vi "Parse Notes.vi"(8 "error in":errorcluster, 11 "String":string) -> (0 "error out":errorcluster, 1 "Done Reading?":bool, 2 "sr note out":string[](array[string]), 3 "result string out":string)   [LabVIEW 2018]
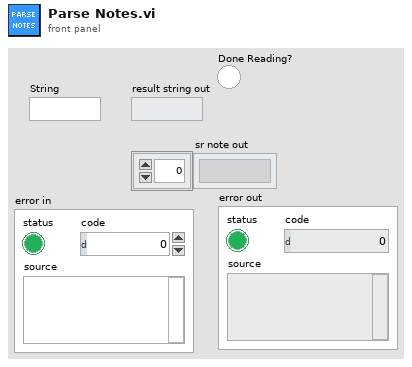
[diagram p1: front panel]
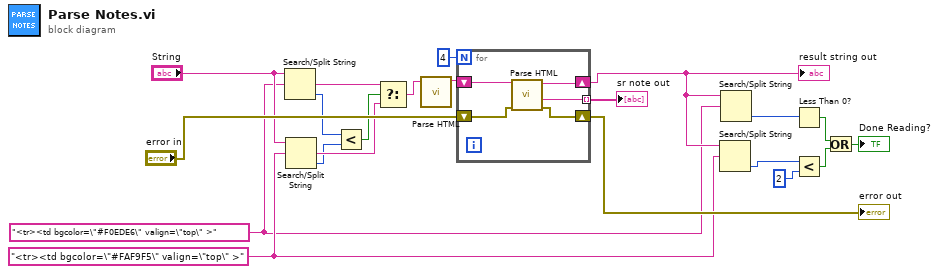
[diagram p0: block diagram]
diagram:
  w6 = "<tr><td bgcolor=\"#FAF9F5\" valign=\"top\" >" ("search string/char (-)")
  w4 = "<tr><td bgcolor=\"#F0EDE6\" valign=\"top\" >" ("search string/char (-)")
  n1 = Search/Split String(string="String", search string/char (-)=w4) -> (match + rest of string=w15:string, offset of match=w13:i32)  [unwired: 1 in, 1 out]
  n2 = Search/Split String(string="String", search string/char (-)=w6) -> (match + rest of string=w14:string, offset of match=w12:i32)  [unwired: 1 in, 1 out]
  n3 = Less?(x=w13, y=w12) -> (x < y?=w11:bool)
  n4 = Select(t=w15, s=w11, f=w14) -> (s? t:f=w3:string)
  n5 = call "Parse HTML.vi"("result string in"=w3) -> ("result string out"=w19:string)  [unwired: 8 in, 2 out]
  n6 = for {
    N: 4 -> [_]
    shift-right: [w25] -> w5
    shift-left: w19 -> [w26]
    tunnel: [w24] -> w21 mode=indexing
    shift-right: [w22] -> w16
    shift-left: "error in" -> [w23]
    n7 = call "Parse HTML.vi"("error in"=w23, "result string in"=w26) -> ("error out"=w22:errorcluster, "data"=w24:string, "result string out"=w25:string)  [unwired: 7 in]
  }
  "result string out" <- w5
  "sr note out" <- w21
  "error out" <- w16
  n8 = Search/Split String(string=w5, search string/char (-)=w6) -> (offset of match=w1:i32)  [unwired: 1 in, 2 out]
  n9 = Search/Split String(string=w5, search string/char (-)=w4) -> (offset of match=w18:i32)  [unwired: 1 in, 2 out]
  n10 = Less Than 0?(x=w18) -> (x < 0?=w8:bool)
  n11 = Less?(x=w1, y=2) -> (x < y?=w9:bool)
  n12 = Or(x=w8, y=w9) -> (x .or. y?=→"Done Reading?":bool)
